vi "Update Delays.vi"(8 "error in (no error)":errorcluster, 10 "BME_DG_Chnl in":refnum<class "BME_DG_Chnl.lvclass">, 11 "BME_DG_System in":refnum<class "BME_DG_System.lvclass">) -> (0 "error out":errorcluster, 3 "BME_DG_System out":refnum<class "BME_DG_System.lvclass">)   [LabVIEW 2009, in "BME_DG_System.lvclass"]
uses:
  BME_DG_System.lvclass
  BME_DG_Chnl/BME_DG_Chnl.lvclass
  BME_DG_System.lvclass/BME_DG_System.ctl
  BME_DG_Base/BME_DG_Base.lvclass
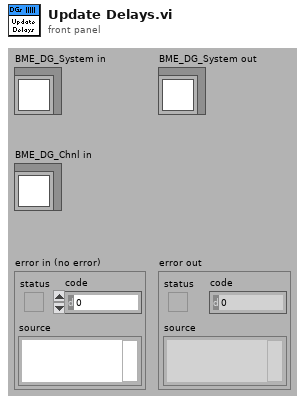
[diagram p1: front panel]
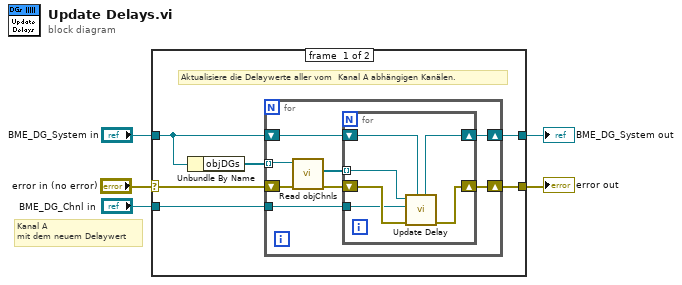
[diagram p0: block diagram]
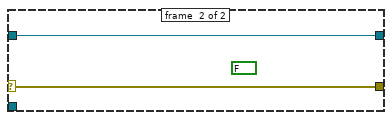
[diagram p2: hidden frame]
diagram:
  # "Kanal A\nmit dem neuem Delaywert"
  n1 = case shown="No Error" "error in (no error)" {
    selector: "error in (no error)" -> [w9 w27]
    tunnel: [w8 w27] -> w4
    tunnel: [w6 w26] -> w2
    tunnel: "BME_DG_System in" -> [w10 w26]
    tunnel: "BME_DG_Chnl in" -> [w7 _]
    frame #0 {
      # "Aktualisiere die Delaywerte aller vom  Kanal A abhängigen Kanälen."
      n2 = Unbundle By Name(w10) -> ("objDGs"=w11:refnum<class "BME_DG_Base.lvclass">[])
      n3 = for {
        tunnel: w11 -> [w19] mode=indexing
        shift-right: [w13] -> w6
        shift-left: w10 -> [w17]
        shift-right: [w12] -> w8
        shift-left: w9 -> [w16]
        tunnel: w7 -> [w14]
        n4 = call-dynamic "Read objChnls.vi"("error in (no error)"=w16, "BME_DG_Base in"=w19) -> ("error out"=w15:errorcluster, "objChnls"=w18:refnum<class "BME_DG_Chnl.lvclass">[])  [unwired: 6 in, 2 out]
        n5 = for {
          tunnel: w18 -> [w25] mode=indexing
          shift-right: [w21] -> w13
          shift-left: w17 -> [w22]
          shift-right: [w23] -> w12
          shift-left: w15 -> [w24]
          tunnel: w14 -> [w20]
          n6 = call "Update Delay.vi"("BME_DG_System"=w22, "error in (no error)"=w24, "Chnl A"=w20, "Chnl2Change"=w25) -> ("error out"=w23:errorcluster, "BME_DG_System out"=w21:refnum<class "BME_DG_System.lvclass">)  [unwired: 6 in]
        }
      }
    }
    frame #1 {
      (unwired) FALSE
    }
  }
  "error out" <- w4
  "BME_DG_System out" <- w2
